vi "Configure Bus Threshold.vi"(6 "Lower Threshold (0 V)":dbl, 7 "Upper Threshold (0 V)":dbl, 8 "error in (no error)":errorcluster, 10 "Channel (0: Channel 1)":u16(ring) items=["Channel 1", "Channel 2", "Channel 3", "Channel 4", "Math", "Reference 1", "Reference 2", "Reference 3", "Reference 4"], 11 "VISA resource name":refnum<visa-resource-name>) -> (0 "error out":errorcluster, 3 "VISA resource name out":refnum<visa-resource-name>)   [LabVIEW 2017, in "Scope.lvlib" / "Tektronix DPO MSO 2000 4000 Series.lvlib"]
doc: "Configures the bus thresholds settings. \n\n<B>Note:</B>\nThis VI only applies to DPO/MSO 4kB, MDO 3000 models."
uses:
  Tektronix DPO MSO 2000 4000 Series.lvlib
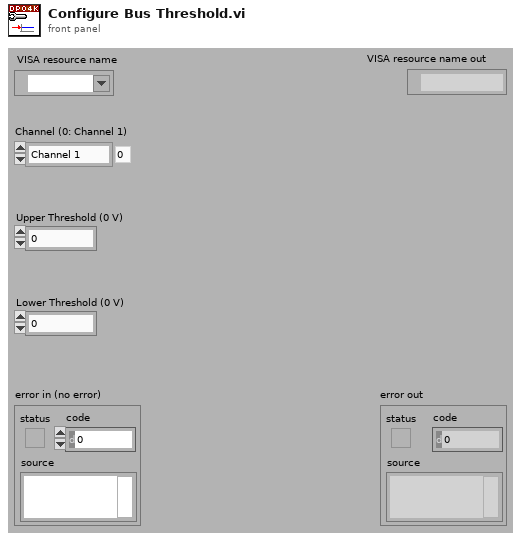
[diagram p1: front panel]
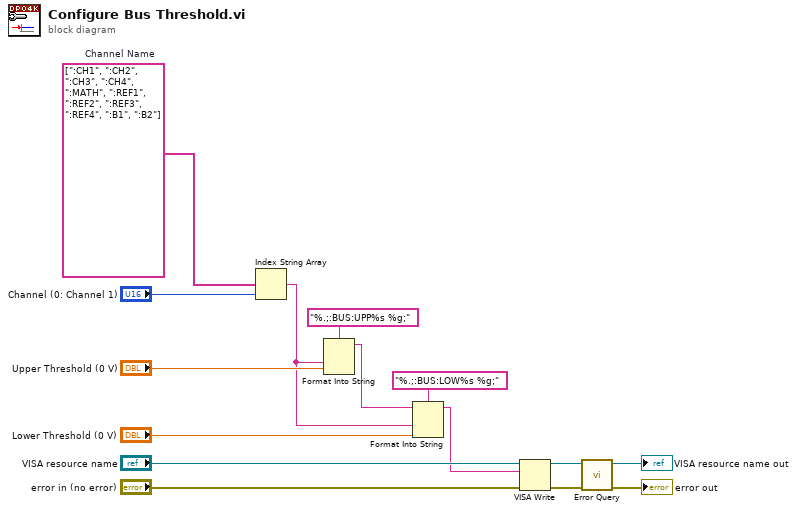
[diagram p0: block diagram]
diagram:
  w9 = string[] [":CH1", ":CH2", ":CH3", ":CH4", ":MATH", ":REF1", ":REF2", ":REF3", ":REF4", ":B1", ":B2"]  # Channel Name
  n1 = Index String Array(1:"Channel (0: Channel 1)", 2:w9) -> (0:w2:string)  [unwired: 1 in]
  n2 = Format Into String(format string="%.;:BUS:UPP%s %g;", w2, "Upper Threshold (0 V)") -> (resulting string=w4:string)  [unwired: 2 in, 1 out]
  n3 = Format Into String(format string="%.;:BUS:LOW%s %g;", initial string=w4, w2, "Lower Threshold (0 V)") -> (resulting string=w1:string)  [unwired: 1 in, 1 out]
  n4 = VISA Write(VISA resource name="VISA resource name", write buffer=w1, error in (no error)="error in (no error)") -> (VISA resource name out=w13:refnum<visa-resource-name>, error out=w12:errorcluster)  [unwired: 1 out]
  n5 = call "Error Query.vi"("error in (no error)"=w12, "VISA resource name"=w13) -> ("error out"=→"error out":errorcluster, "VISA resource name out"=→"VISA resource name out":refnum<visa-resource-name>)  [unwired: 6 in, 2 out]
